vi "Pack for gRPC.vi"(8 "error in (no error)":errorcluster, 9 "Configuration / Resuls (Config)":enum16{"Configuration", "Results"}(ring), 10 "Data Value":variant, 11 "Measurement Customizations in":refnum<class "MeasurementPlugin.lvclass">) -> (0 "error out":errorcluster, 2 "Any":T1, 3 "Measurement Customizations out":refnum<class "MeasurementPlugin.lvclass">)   [LabVIEW 2021, in "Crosstalk Sweep.lvlib" / "MeasurementPlugin.lvclass"]
uses:
  MeasurementPlugin.lvclass
  <vilib>/gRPC/LabVIEW gRPC Library/Shared/Any.ctl
  C:/Program Files/National Instruments/LabVIEW 2021/vi.lib/MeasurementLink/MeasurementLink Measurement Server/Measurement Plugin Service/Measurement Plugin Service.lvclass
  Measurement Configuration.ctl
  shared/controls/digital output level units.ctl
  shared/controls/weighting filter.ctl
  shared/controls/highpass filter.ctl
  shared/controls/lowpass filter.ctl
  Measurement Results.ctl
  2eca732d-dbaa-43bf-a7dd-ede2da65bc1b.vi
  a6012965-5700-4384-8228-972e71b6560c.vi
  <vilib>/gRPC/LabVIEW gRPC Library/Server API/Translate Protobuf Error.vi
  <vilib>/AdvancedString/1D String Array to Delimited String.vi
  <vilib>/gRPC/LabVIEW gRPC Library/Server API/Server/Get Server DLL Path.vi
  MeasurementPlugin.lvclass/MeasurementPlugin.ctl
  Crosstalk Sweep.lvlib
  <vilib>/MeasurementLink/MeasurementLink Measurement Server/Measurement Plugin Service/Measurement Plugin Service.lvclass
  shared/controls/audio controls.lvlib
  shared/controls/sweep profile.ctl
  <vilib>/gRPC/LabVIEW gRPC Library/grpc-lvsupport-release.lvlib
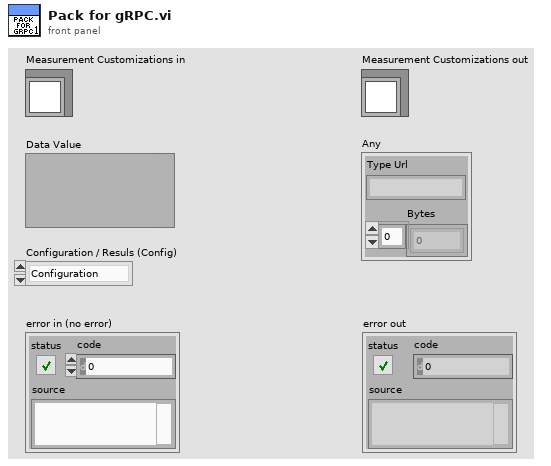
[diagram p1: front panel]
types:
  T1 = typedef "grpc-lvsupport-release.lvlib/Any.ctl" = cluster{"Type Url":string, "Bytes":u8[]}
  T2 = typedef "grpc-lvsupport-release.lvlib/grpcId.ctl" = u64
  T3 = typedef "Crosstalk Sweep.lvlib/Measurement Configuration.ctl" = cluster{"digital serial cfg file":string, "digital channel list":string, "master clock channel list":string, "digital audio interferrer channel":i32, "output level":dbl, "output level units":T4, "output range (pk-pk)":dbl, "load impedance":dbl, "acq channel - victim":string, "acq channel - interferrer":string, "acq sampling rate":dbl, "sweep start frequency (Hz)":dbl, "sweep stop frequency (Hz)":dbl, "number of steps":u32, "sweep profile":T5, "min measurement cycles":u32, "min measurement time (s)":dbl, "min settling cycles":u32, "min settling time (s)":dbl, "band start":dbl, "band stop":dbl, "weighting filter":T6, "highpass filter":T7, "lowpass filter":T8}
  T4 = typedef "audio controls.lvlib/digital output level units.ctl" = enum32{"% FS", "dBFS", "V"}
  T5 = typedef "audio controls.lvlib/sweep profile.ctl" = enum32{"Linear", "Logarithmic"}
  T6 = typedef "weighting filter.ctl" = enum32{"Linear", "A-weighting", "B-weighting", "C-weighting"}
  T7 = typedef "highpass filter.ctl" = enum32{"DC", "AC"}
  T8 = typedef "lowpass filter.ctl" = enum32{"No filter", "AES17 20kHz", "AES17 40kHz"}
  T9 = typedef "Crosstalk Sweep.lvlib/Measurement Results.ctl" = cluster{"channel names":string[], "frequency (Hz)":dbl[], "crosstalk (dB)":dbl[], "wfm - t0":dbl, "wfm - dt":dbl, "wfm - data":dbl[], "fft - f0":dbl, "fft - df":dbl, "fft - data":dbl[]}
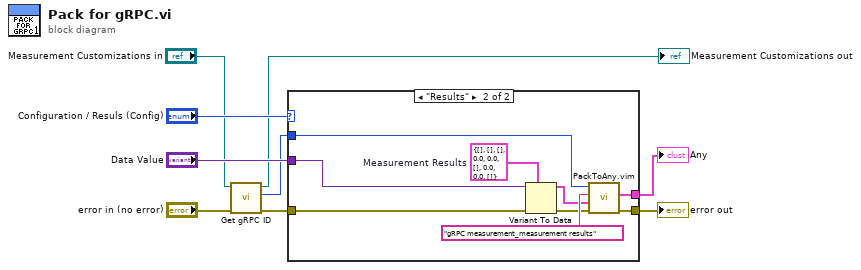
[diagram p0: block diagram]
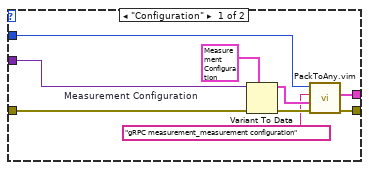
[diagram p2: hidden frame]
diagram:
  n1 = call <vilib>:"Get gRPC ID.vi"("error in"="error in (no error)", "measurement plugin service in"="Measurement Customizations in") -> ("error out"=w4:errorcluster, "gRPC ID"=w1:T2, "measurement plugin service out"=→"Measurement Customizations out":refnum<class "MeasurementPlugin.lvclass">)  [unwired: 7 in]
  n2 = case shown="\"Results\"" "Configuration / Resuls (Config)" {
    tunnel: w4 -> [w18 w27]
    tunnel: "Data Value" -> [w17 w26]
    tunnel: w1 -> [w14 w22]
    tunnel: [w16 w24] -> w8
    tunnel: [w15 w23] -> w7
    frame "Configuration" {
      w11 = T3 {"digital serial cfg file"="", "digital channel list"="7821\\PCMo 8", "master clock channel list"="7821\\PCMo 0", "digital audio interferrer channel"=0, "output level"=20.0, "output level units"=enum."dBFS", "output range (pk-pk)"=3.16, "load impedance"=4.0, "acq channel - victim"="", "acq channel - interferrer"="", "acq sampling rate"=1000.0, "sweep start frequency (Hz)"=20000.0, "sweep stop frequency (Hz)"=0.0, "number of steps"=0, "sweep profile"=enum."Linear", "min measurement cycles"=1000, "min measurement time (s)"=5.0, "min settling cycles"=0, "min settling time (s)"=5.0, "band start"=20.0, "band stop"=20000.0, "weighting filter"=enum."Linear", "highpass filter"=enum."DC", "lowpass filter"=enum."No filter"}  # Measurement Configuration
      n3 = Variant To Data(error in=w18, type=w11, Variant=w17) -> (data=w13:T3, error out=w12:errorcluster)
      n4 = call "PackToAny.vim"("error in"=w12, "Data To Pack"=w13, "Message Type"="gRPC measurement_measurement configuration", "gRPCid in"=w14) -> ("error out"=w16:errorcluster, "Any"=w15:T1)  [unwired: 5 in, 1 out]
    }
    frame "Results" {
      w25 = T9 {"channel names"=[], "frequency (Hz)"=[], "crosstalk (dB)"=[], "wfm - t0"=0.0, "wfm - dt"=0.0, "wfm - data"=[], "fft - f0"=0.0, "fft - df"=0.0, "fft - data"=[]}  # Measurement Results
      n5 = Variant To Data(error in=w27, type=w25, Variant=w26) -> (data=w20:T9, error out=w19:errorcluster)
      n6 = call "PackToAny.vim"("error in"=w19, "Data To Pack"=w20, "Message Type"="gRPC measurement_measurement results", "gRPCid in"=w22) -> ("error out"=w24:errorcluster, "Any"=w23:T1)  [unwired: 5 in, 1 out]
    }
  }
  "error out" <- w8
  "Any" <- w7
